vi "Discover_Gantry_TestBench.vi"(0 "Session In":refnum<visa-resource-name>="COM5", 5 "error in":errorcluster {"code" format="%.0x"}, 9 "Close Session(t)":bool=TRUE) -> (10 "Gantry Present(t)":bool=TRUE, 12 "TestBench_ID":string="WAM_PROD_TEST-1", 13 "concatenated string":string="#INST: Gantry#Address COM5#Manufacturer Zaber#Model X-MCC4 (rev 1)#SN 81246#Ver (FW) 7.21 (DR) 1.5", 14 "Session Out":refnum<visa-resource-name>="COM5", 15 "Mfr":string="Zaber", 16 "Model":string="X-MCC4 (rev 1)", 17 "Ver":string="(FW) 7.21 (DR) 1.5", 18 "SN":string="81246", 19 "error out":errorcluster)   [LabVIEW 2018]
uses:
  Instruments/Zaber Gantry/Zaber Labview Driver/Zaber A Series.lvlib
  Initialize References/Sequence Globals.vi
  <vilib>/Utility/file.llb/Read Delimited Spreadsheet (string).vi
panel:
  out "FH_NOT(T)":bool=TRUE
  out "S/N":string="81246"
  out "Instrument Driver Revision":string="1.5"
  out "Instrument Firmware Revision":string="7.21"
  out "Pass Self-Test(t)":bool=TRUE
  out "Peripheral ID":i32=70140
  out "Device ID":i32=30342
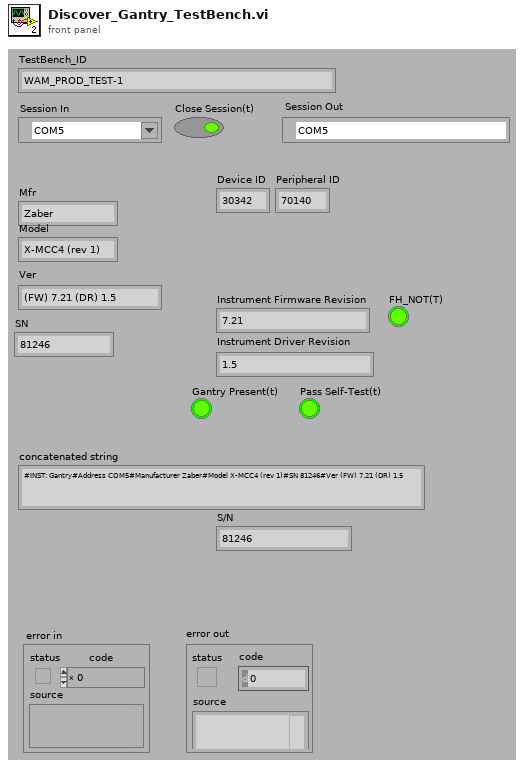
[diagram p1: front panel]
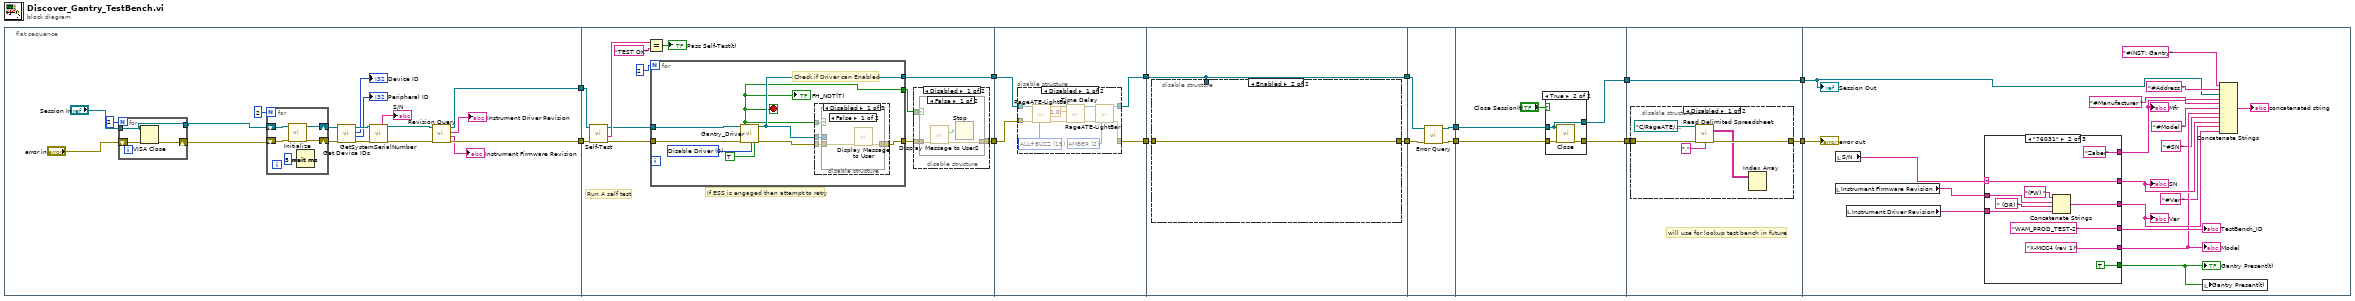
[diagram p0: block diagram]
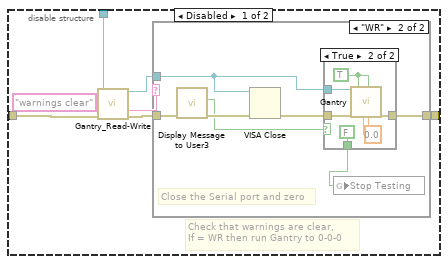
[diagram p7: hidden frame]
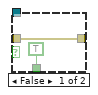
[diagram p9: hidden frame]
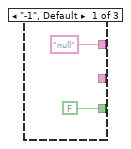
[diagram p12: hidden frame]
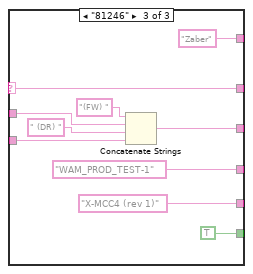
[diagram p13: hidden frame]
diagram:
  n1 = flat-sequence {
    tunnel: [w24] -> w14
    tunnel: [w21] -> w13
    tunnel: w14 -> [w42]
    tunnel: w13 -> [w43]
    tunnel: [w47] -> w8
    tunnel: [w45] -> w6
    tunnel: w8 -> [w79]
    tunnel: [w78] -> w7
    tunnel: w6 -> [w80]
    tunnel: [w81] -> w5
    tunnel: w7 -> [w94]
    tunnel: w5 -> [w96]
    tunnel: [w95] -> w12
    tunnel: [w94] -> w11
    tunnel: [w123] -> w10
    tunnel: [w122] -> w9
    tunnel: w12 -> [w124]
    tunnel: w11 -> [w121]
    tunnel: [w128] -> w4
    tunnel: [w127] -> w2
    tunnel: w9 -> [w125]
    tunnel: w10 -> [w126]
    tunnel: w4 -> [w135]
    tunnel: [w136] -> w3
    tunnel: w2 -> [w137]
    tunnel: [w137] -> w1
    tunnel: w3 -> [w146]
    tunnel: w1 -> [w145]
    frame #0 {
      n2 = for {
        N: 2 -> [_]
        tunnel: "Session In" -> [w34]
        shift-right: [w35] -> w17
        shift-left: "error in" -> [w36]
        tunnel: [w34] -> w15
        n3 = VISA Close(VISA resource name=w34, error in (no error)=w36) -> (error out=w35:errorcluster)
      }
      n4 = for {
        N: 2 -> [_]
        shift-right: [w40] -> w30
        shift-left: w15 -> [w39]
        shift-right: [w41] -> w31
        shift-left: w17 -> [w38]
        n5 = call "Initialize.vi"("error in (no error)"=w38, "VISA resource name"=w39) -> ("error out"=w41:errorcluster, "VISA resource name out"=w40:refnum<visa-resource-name>)  [unwired: 8 in]
        n6 = Wait (ms)(milliseconds to wait=u32 5) -> ()  [unwired: 1 out]
      }
      n7 = call "Get Device IDs.vi"("error in (no error)"=w31, "VISA resource name"=w30) -> ("error out"=w33:errorcluster, "Peripheral ID"=→"Peripheral ID":i32, "Device ID"=→"Device ID":i32, "VISA resource name out"=w32:refnum<visa-resource-name>)  [unwired: 6 in]
      n8 = call "GetSystemSerialNumber.vi"("VISA resource name"=w32, "error in (no error)"=w33) -> ("S/N"=→"S/N":string, "VISA resource name out"=w25:refnum<visa-resource-name>, "error out"=w26:errorcluster)  [unwired: 11 in]
      n9 = call "Revision Query.vi"("error in (no error)"=w26, "VISA resource name"=w25) -> ("error out"=w24:errorcluster, "Instrument Firmware Revision"=→"Instrument Firmware Revision":string, "Instrument Driver Revision"=→"Instrument Driver Revision":string, "VISA resource name out"=w21:refnum<visa-resource-name>)  [unwired: 6 in]
    }
    frame #1 {
      # "If ESS is engaged then attempt to retry"
      # "Run A self test"
      n10 = call "Self-Test.vi"("error in (no error)"=w42, "VISA resource name"=w43) -> ("error out"=w50:errorcluster, "Self-Test Result Message"=w51:string, "VISA resource name out"=w49:refnum<visa-resource-name>)  [unwired: 7 in]
      n11 = Equal?(x=w51, y="TEST OK") -> (x = y?=→"Pass Self-Test(t)":bool)
      n12 = for {
        N: 2 -> [_]
        tunnel: w50 -> [w69]
        tunnel: w49 -> [w68]
        tunnel: [w65] -> w46
        tunnel: [w64] -> w47
        tunnel: [w63] -> w44
        stop <- w63 stop-if-true
        w67 = u16 0 items=["Disable Driver", "Enable Driver", "Read Driver Status"] ("Driver-Func")
        # "Check if Driver can Enabled"
        n13 = call "Gantry_Driver.vi"("VISA resource name"=w68, "error in (no error)"=w69, "Driver-Func"=w67, "Close Serial"=TRUE) -> ("FH_NOT(T)"=w63:bool, "VISA resource name out"=w64:refnum<visa-resource-name>, "error out"=w66:errorcluster)  [unwired: 12 in, 1 out]
        "FH_NOT(T)" <- w63
        n14 = disable-structure shown="Disabled" {
          disable-tunnel: w66 -> [w73 w77]
          disable-tunnel: [w72 w77] -> w65
          disable-tunnel: w64 -> [w71 _]
          disable-tunnel: w63 -> [w70 _]
          frame Disabled {
            n15 = case shown="False" w70 {
              tunnel: w71 -> [_ _]
              tunnel: w73 -> [w74 w76]
              tunnel: [w75 w76] -> w72
              frame False {
                n16 = call "Display Message to User"("error in (no error)"=w74) -> ("error out"=w75:errorcluster)  [unwired: 9 in, 1 out]
              }
              frame True {
              }
            }
          }
          frame Enabled {
          }
        }
      }
      n17 = disable-structure shown="Disabled" {
        disable-tunnel: w46 -> [w56 w61]
        disable-tunnel: [w55 w61] -> w45
        disable-tunnel: w44 -> [w54 _]
        frame Disabled {
          n18 = case shown="False" w54 {
            tunnel: w56 -> [w59 w60]
            tunnel: [w58 w60] -> w55
            frame False {
              n19 = call "Display Message to User2"("error in (no error)"=w59) -> ("error out"=w58:errorcluster, "OK"=w57:bool)  [unwired: 9 in]
              n20 = Stop(stop? (T)=w57) -> ()
            }
            frame True {
            }
          }
        }
        frame Enabled {
        }
      }
    }
    frame #2 {
      n21 = disable-structure shown="Disabled" {
        disable-tunnel: [w91 w92] -> w81
        disable-tunnel: w80 -> [w90 w92]
        disable-tunnel: w79 -> [w89 w93]
        disable-tunnel: [w88 w93] -> w78
        frame Disabled {
          w86 = u32 2 items=["RED"=1, "AMBER"=2, "GREEN"=4, "ALL"=7, "BUZZ"=8, "RED+BUZZ"=9, "ALL+BUZZ"=15] ("Select")
          w87 = u32 15 items=["RED"=1, "AMBER"=2, "GREEN"=4, "ALL"=7, "BUZZ"=8, "RED+BUZZ"=9, "ALL+BUZZ"=15] ("Select")
          n22 = call "RageATE-LightBar.vi"("VISA resource name"=w89, "error in"=w90, "Select"=w87) -> ("VISA resource name out"=w85:refnum<visa-resource-name>, "error out"=w83:errorcluster)  [unwired: 10 in, 1 out]
          n23 = call "Time Delay"("error in (no error)"=w83, "Delay Time (s)"=1.0) -> ("error out"=w84:errorcluster)  [unwired: 9 in]
          n24 = call "RageATE-LightBar.vi"("VISA resource name"=w85, "error in"=w84, "Select"=w86) -> ("VISA resource name out"=w88:refnum<visa-resource-name>, "error out"=w91:errorcluster)  [unwired: 10 in, 1 out]
        }
        frame Enabled {
        }
      }
    }
    frame #3 {
      n25 = disable-structure shown="Enabled" {
        disable-tunnel: w96 -> [w102 w120]
        disable-tunnel: [w98 w120] -> w95
        disable-tunnel: w94 -> [w97 _]
        frame Disabled {
          # "Check that warnings are clear,\nIf = WR then run Gantry to 0-0-0"
          n26 = call "Gantry_Read-Write.vi"("VISA resource name"=w97, "Command"="warnings clear", "error in (no error)"=w102) -> ("VISA resource name out"=w99:refnum<visa-resource-name>, "Warning Flags"=w101:string, "error out"=w100:errorcluster)  [unwired: 6 in, 4 out]
          n27 = case shown="\"WR\"" w101 {
            tunnel: w100 -> [w104 w107]
            tunnel: w99 -> [_ w110]
            tunnel: [w104 w111] -> w98
            frame "False", Default {
            }
            frame "WR" {
              # "Close the Serial port and zero"
              n28 = call "Display Message to User3"("error in (no error)"=w107) -> ("error out"=w108:errorcluster, "OK"=w106:bool)  [unwired: 9 in]
              n29 = VISA Close(VISA resource name=w110, error in (no error)=w108) -> (error out=w109:errorcluster)
              n30 = case shown="True" w106 {
                tunnel: [w113 w119] -> w111
                tunnel: w110 -> [_ w116]
                tunnel: w109 -> [w113 w115]
                tunnel: [TRUE ("Stop Testing") FALSE ("Stop Testing")] -> w105
                frame False {
                }
                frame True {
                  w118 = 0.0 ("z ref")
                  w117 = TRUE ("Use manual(t)")
                  n31 = call "Gantry.vi"("COMPORT"=w116, "error in (no error)"=w115, "Use manual(t)"=w117, "z ref"=w118, "Write(reads antenna co-ords when off)"=w117, "z"=w118) -> ("error out"=w119:errorcluster)  [unwired: 13 in]
                }
              }
              n32 = global write "Sequence Globals.vi" "Stop Testing"(w105) -> ()
            }
          }
        }
        frame Enabled {
        }
      }
    }
    frame #4 {
      n33 = call "Error Query.vi"("error in (no error)"=w124, "VISA resource name"=w121) -> ("error out"=w123:errorcluster, "VISA resource name out"=w122:refnum<visa-resource-name>)  [unwired: 6 in, 2 out]
    }
    frame #5 {
      n34 = case shown="True" "Close Session(t)" {
        tunnel: w126 -> [w131 w134]
        tunnel: [w131 w133] -> w128
        tunnel: w125 -> [w130 w132]
        tunnel: [w130 w132] -> w127
        frame False {
        }
        frame True {
          n35 = call "Close.vi"("error in (no error)"=w134, "VISA resource name"=w132) -> ("error out"=w133:errorcluster)  [unwired: 9 in]
        }
      }
    }
    frame #6 {
      # "will use for lookup test bench in future"
      n36 = disable-structure shown="Disabled" {
        disable-tunnel: [w142 w143] -> w136
        disable-tunnel: w135 -> [w141 w143]
        frame Disabled {
          n37 = call-poly <vilib>:"Read Delimited Spreadsheet.vi"("file path (dialog if empty)"=path "C:/RageATE/Automated Tests/Tetra WAM/PRODUCTION/setup files/TestBenches.txt", "error in (no error)"=w141, "delimiter (\\t)"="," ("delimiter (\\t)")) -> ("all rows"=w139:string[][], "error out"=w142:errorcluster)  [unwired: 7 in, 4 out]
          n38 = Index Array(array=w139) -> ()  [unwired: 2 in, 1 out]
        }
        frame Enabled {
        }
      }
    }
    frame #7 {
      n39 = local read "Instrument Firmware Revision"() -> (w160:string)
      n40 = local read "S/N"() -> (w159:string)
      n41 = local read "Instrument Driver Revision"() -> (w161:string)
      n42 = case shown="\"76031\"" w159 {
        selector: w159 -> [_ w164 w174]
        tunnel: [_ "Zaber" ("string") "Zaber" ("string")] -> w154
        tunnel: [_ "X-MCC4 (rev 1)" ("string") "X-MCC4 (rev 1)" ("string")] -> w155
        tunnel: [_ w164 w174] -> w156
        tunnel: [_ w171 w181] -> w153
        tunnel: w160 -> [_ w170 w180]
        tunnel: w161 -> [_ w167 w177]
        tunnel: [FALSE ("Gantry Present(t)") TRUE TRUE] -> w157
        tunnel: ["null" ("string") "WAM_PROD_TEST-2" ("string") "WAM_PROD_TEST-1" ("string")] -> w158
        frame "-1", Default {
        }
        frame "76031" {
          n43 = Concatenate Strings("(FW) " ("string"), w170, " (DR) " ("string"), w167) -> (w171:string)
        }
        frame "81246" {
          n44 = Concatenate Strings("(FW) " ("string"), w180, " (DR) " ("string"), w177) -> (w181:string)
        }
      }
      "Ver" <- w153
      "Mfr" <- w154
      "Model" <- w155
      "SN" <- w156
      "Gantry Present(t)" <- w157
      "TestBench_ID" <- w158
      n45 = local write "Gantry Present(t)"(w157) -> ()
      n46 = Concatenate Strings("#INST: Gantry" ("string"), "#Address " ("string"), w145, "#Manufacturer ", w154, "#Model ", w155, "#SN " ("string"), w156, "#Ver " ("string"), w153) -> (→"concatenated string":string)
      "Session Out" <- w145
      "error out" <- w146
    }
  }
